vi "Cache_Info Load.vi"(0 "Refnum in":T2, 5 "Class Name":string, 11 "error in (no error)":errorcluster) -> (4 "Refnum out":T2, 6 "Class Info":T1, 8 "Is Interface":bool, 10 "Success?":bool, 15 "error out":errorcluster)   [LabVIEW 2020, in "ClassLoader.lvlib"]
uses:
  <vilib>/Utility/config.llb/Config Data RefNum.ctl
  ClassLoader.lvlib
  <vilib>/Utility/config.llb/NI_LVConfig.lvlib
  <vilib>/Utility/config.llb/Read Key (Boolean).vi
  <vilib>/Utility/config.llb/Read Key (String).vi
  Ctl/Ctl_Class Info.ctl
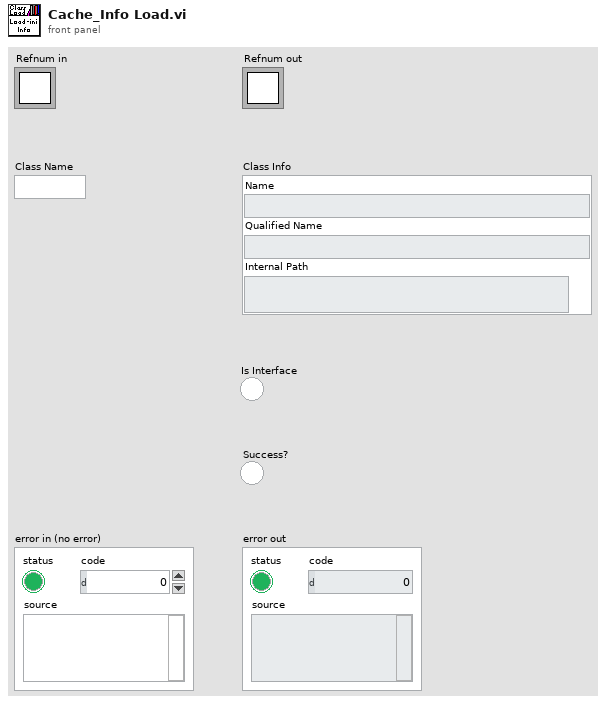
[diagram p1: front panel]
types:
  T1 = typedef "ClassLoader.lvlib/Ctl_Class Info.ctl" = cluster{"Name":string, "Qualified Name":string, "Internal Path":string}
  T2 = typedef "NI_LVConfig.lvlib/Config Data RefNum.ctl" = refnum<k1>
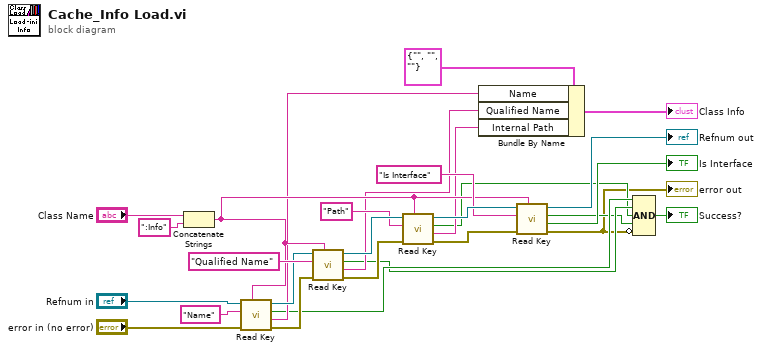
[diagram p0: block diagram]
diagram:
  n1 = Concatenate Strings("Class Name", ":Info" ("string")) -> (w17:string)
  n2 = call-poly <vilib>:"Read Key.vi"("section"=w17, "error in (no error)"="error in (no error)", "key"="Name", "refnum"="Refnum in") -> ("error out"=w26:errorcluster, "value"=w10:string, "found?"=w6:bool, "refnum out"=w24:T2)  [unwired: 4 in]
  n3 = call-poly <vilib>:"Read Key.vi"("section"=w17, "error in (no error)"=w26, "key"="Qualified Name", "refnum"=w24) -> ("error out"=w21:errorcluster, "value"=w9:string, "found?"=w5:bool, "refnum out"=w23:T2)  [unwired: 4 in]
  n4 = call-poly <vilib>:"Read Key.vi"("section"=w17, "error in (no error)"=w21, "key"="Path", "refnum"=w23) -> ("error out"=w18:errorcluster, "value"=w8:string, "found?"=w4:bool, "refnum out"=w20:T2)  [unwired: 4 in]
  n5 = Bundle By Name(cluster=T1 {"Name"="", "Qualified Name"="", "Internal Path"=""} ("Class Info"), "Name"=w10, "Qualified Name"=w9, "Internal Path"=w8) -> (→"Class Info":T1)
  n6 = call-poly <vilib>:"Read Key.vi"("section"=w17, "error in (no error)"=w18, "key"="Is Interface", "refnum"=w20) -> ("error out"=w2:errorcluster, "value"=→"Is Interface":bool, "found?"=w3:bool, "refnum out"=→"Refnum out":T2)  [unwired: 4 in]
  "error out" <- w2
  n7 = Compound Arithmetic op=AND(w6, w5, w4, w3, invert w2) -> (→"Success?":bool)
